vi "change type for single diagram.vi"(8 "error in (no error)":errorcluster, 9 "old type":T1, 10 "new type":T1, 11 "Diagram in":refnum<vi>) -> ()   [LabVIEW 2013]
uses:
  source/tag/Data Type.ctl
  source/tag/tag descriptor.lvclass
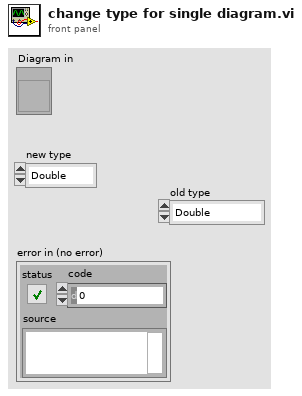
[diagram p1: front panel]
types:
  T1 = typedef "tag bus.lvlib/tag descriptor.lvclass/Data Type.ctl" = enum16{"Double", "Single", "I64", "I32", "I16", "I8", "U64", "U32", "U16", "U8", "Boolean", "String", "Array of Double", "Array of Single", "Array of I64", "Array of I32", "Array of I16", "Array of I8", "Array of U64", "Array of U32", "Array of U16", "Array of U8", "Array of Boolean", "Array of String"}
  T2 = cluster{"VIPath":path, "Menu Name":string, "Selector Name":string}[]
  T3 = cluster{"VIPath":path, "Menu Name":string, "Selector Name":string}
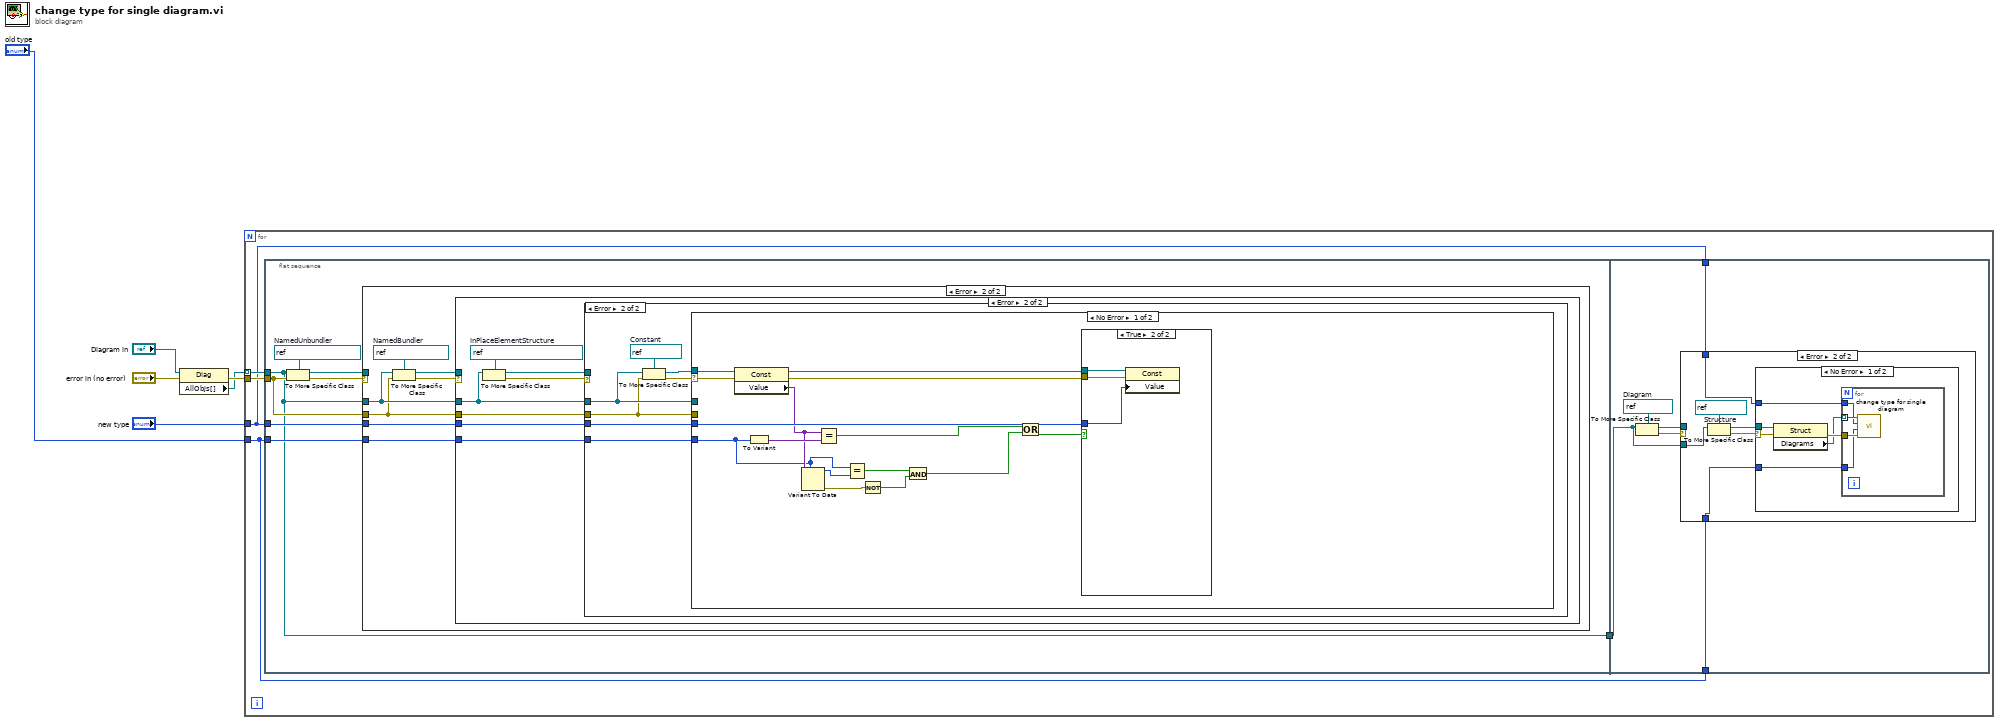
[diagram p0: block diagram]
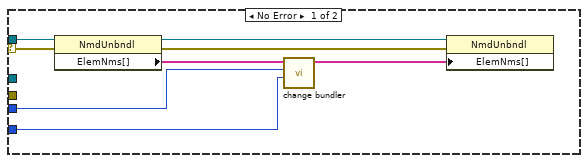
[diagram p2: hidden frame]
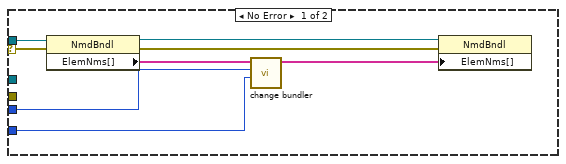
[diagram p3: hidden frame]
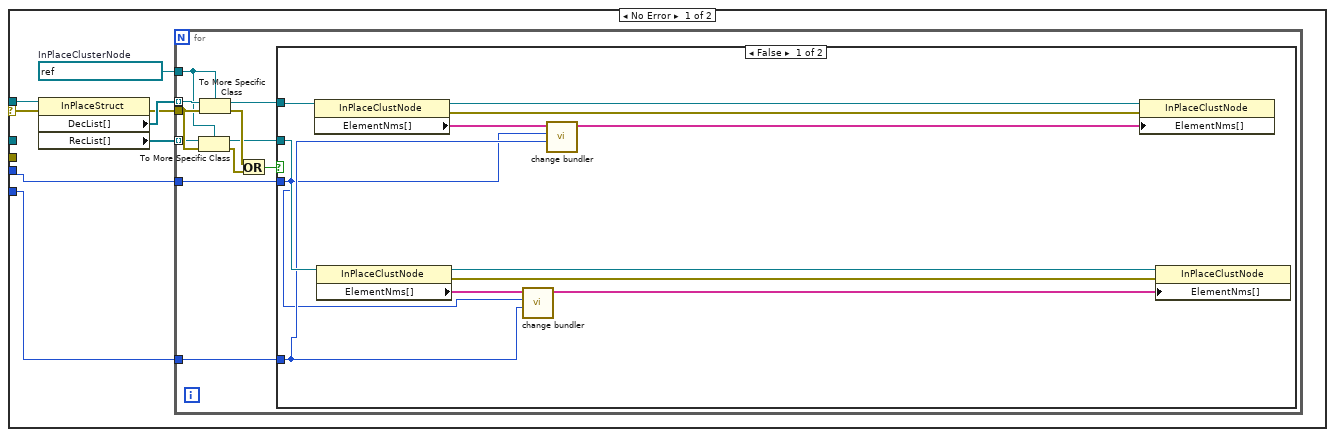
[diagram p4: hidden frame]
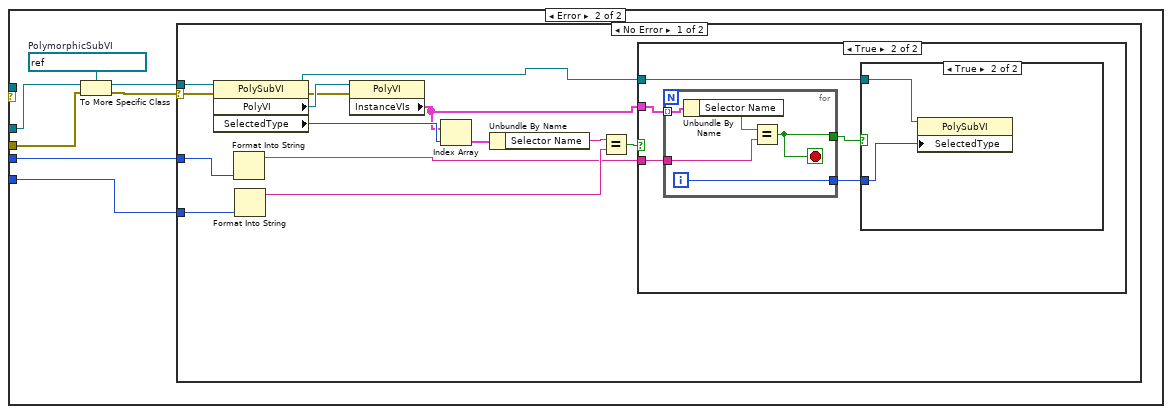
[diagram p7: hidden frame]
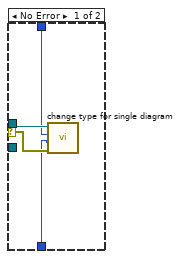
[diagram p11: hidden frame]
diagram:
  n1 = property class="Diag"(reference="Diagram in", error in="error in (no error)") -> (error out=w4:errorcluster, "AllObjs[]"=w3:refnum<vi>[])  [unwired: 1 out]
  n2 = for {
    tunnel: w3 -> [w11] mode=indexing
    tunnel: w4 -> [w10]
    tunnel: "old type" -> [w7]
    tunnel: "new type" -> [w8]
    n3 = flat-sequence {
      tunnel: w11 -> [w12]
      tunnel: w10 -> [w15]
      tunnel: w7 -> [w14]
      tunnel: w8 -> [w13]
      tunnel: [w12] -> w9
      tunnel: w9 -> [w138]
      tunnel: w8 -> [w140]
      tunnel: w7 -> [w139]
      frame #0 {
        w18 = refnum<vi> refnum  # NamedUnbundler
        n4 = To More Specific Class(target class=w18, reference=w12, error in=w15) -> (specific class reference=w16:refnum<vi>, error out=w17:errorcluster)
        n5 = case shown="Error" w17 {
          selector: w17 -> [w25 _]
          tunnel: w16 -> [w26 _]
          tunnel: w12 -> [_ w30]
          tunnel: w15 -> [_ w29]
          tunnel: w14 -> [w20 w28]
          tunnel: w13 -> [w19 w27]
          frame No Error {
            n6 = property class="NmdUnbndl"(reference=w26, error in=w25) -> (reference out=w24:refnum<vi>, error out=w23:errorcluster, "ElemNms[]"=w22:string[])
            n7 = call "change bundler.vi"("old data type"=w20, "new data type"=w19, "ElemNms[]"=w22) -> ("elemnames out"=w21:string[])  [unwired: 8 in]
            n8 = property class="NmdUnbndl"(reference=w24, error in=w23, "ElemNms[]"=w21) -> ()  [unwired: 2 out]
          }
          frame Error {
            w33 = refnum<vi> refnum  # NamedBundler
            n9 = To More Specific Class(target class=w33, reference=w30, error in=w29) -> (specific class reference=w31:refnum<vi>, error out=w32:errorcluster)
            n10 = case shown="Error" w32 {
              selector: w32 -> [w36 _]
              tunnel: w31 -> [w37 _]
              tunnel: w30 -> [_ w42]
              tunnel: w29 -> [_ w45]
              tunnel: w28 -> [w34 w44]
              tunnel: w27 -> [w35 w43]
              frame No Error {
                n11 = property class="NmdBndl"(reference=w37, error in=w36) -> (reference out=w40:refnum<vi>, error out=w39:errorcluster, "ElemNms[]"=w41:string[])
                n12 = call "change bundler.vi"("old data type"=w34, "new data type"=w35, "ElemNms[]"=w41) -> ("elemnames out"=w38:string[])  [unwired: 8 in]
                n13 = property class="NmdBndl"(reference=w40, error in=w39, "ElemNms[]"=w38) -> ()  [unwired: 2 out]
              }
              frame Error {
                w48 = refnum<vi> refnum  # InPlaceElementStructure
                n14 = To More Specific Class(target class=w48, reference=w42) -> (specific class reference=w46:refnum<vi>, error out=w47:errorcluster)  [unwired: 1 in]
                n15 = case shown="Error" w47 {
                  selector: w47 -> [w55 _]
                  tunnel: w46 -> [w56 _]
                  tunnel: w42 -> [_ w81]
                  tunnel: w45 -> [_ w80]
                  tunnel: w44 -> [w49 w83]
                  tunnel: w43 -> [w50 w82]
                  frame No Error {
                    w52 = refnum<vi> refnum  # InPlaceClusterNode
                    n16 = property class="InPlaceStruct"(reference=w56, error in=w55) -> (error out=w53:errorcluster, "DecList[]"=w54:refnum<vi>[], "RecList[]"=w51:refnum<vi>[])  [unwired: 1 out]
                    n17 = for {
                      tunnel: w54 -> [w67] mode=indexing
                      tunnel: w53 -> [w66]
                      tunnel: w52 -> [w64]
                      tunnel: w51 -> [w65] mode=indexing
                      tunnel: w50 -> [w58]
                      tunnel: w49 -> [w57]
                      n18 = To More Specific Class(target class=w64, reference=w65, error in=w66) -> (specific class reference=w59:refnum<vi>, error out=w62:errorcluster)
                      n19 = To More Specific Class(target class=w64, reference=w67, error in=w66) -> (specific class reference=w60:refnum<vi>, error out=w63:errorcluster)
                      n20 = Or(x=w63, y=w62) -> (x .or. y?=w61:bool)
                      n21 = case shown="False" w61 {
                        tunnel: w60 -> [w74 _]
                        tunnel: w59 -> [w75 _]
                        tunnel: w58 -> [w68 _]
                        tunnel: w57 -> [w69 _]
                        frame False {
                          n22 = property class="InPlaceClustNode"(reference=w74) -> (reference out=w79:refnum<vi>, error out=w78:errorcluster, "ElementNms[]"=w71:string[])  [unwired: 1 in]
                          n23 = property class="InPlaceClustNode"(reference=w75) -> (reference out=w76:refnum<vi>, error out=w77:errorcluster, "ElementNms[]"=w73:string[])  [unwired: 1 in]
                          n24 = call "change bundler.vi"("old data type"=w69, "new data type"=w68, "ElemNms[]"=w73) -> ("elemnames out"=w72:string[])  [unwired: 8 in]
                          n25 = call "change bundler.vi"("old data type"=w69, "new data type"=w68, "ElemNms[]"=w71) -> ("elemnames out"=w70:string[])  [unwired: 8 in]
                          n26 = property class="InPlaceClustNode"(reference=w79, error in=w78, "ElementNms[]"=w70) -> ()  [unwired: 2 out]
                          n27 = property class="InPlaceClustNode"(reference=w76, error in=w77, "ElementNms[]"=w72) -> ()  [unwired: 2 out]
                        }
                        frame True {
                          # "shouldnt ever happen if I understand ipestructs"
                        }
                      }
                    }
                  }
                  frame Error {
                    w86 = refnum<vi> refnum  # Constant
                    n28 = To More Specific Class(target class=w86, reference=w81, error in=w80) -> (specific class reference=w84:refnum<vi>, error out=w85:errorcluster)
                    n29 = case shown="No Error" w85 {
                      selector: w85 -> [w100 _]
                      tunnel: w84 -> [w101 _]
                      tunnel: w83 -> [w92 w105]
                      tunnel: w82 -> [w95 w106]
                      tunnel: w81 -> [_ w109]
                      tunnel: w80 -> [_ w110]
                      frame No Error {
                        n30 = property class="Const"(reference=w101, error in=w100) -> (reference out=w97:refnum<vi>, error out=w96:errorcluster, "Value"=w94:variant)
                        n31 = To Variant(anything=w92) -> (Variant=w99:variant)
                        n32 = Variant To Data(type=w92, Variant=w94) -> (data=w93:T1, error out=w90:errorcluster)  [unwired: 1 in]
                        n33 = Equal?(x=w94, y=w99) -> (x = y?=w98:bool)
                        n34 = Equal?(x=w92, y=w93) -> (x = y?=w91:bool)
                        n35 = Not(x=w90) -> (.not. x?=w89:bool)
                        n36 = And(x=w91, y=w89) -> (x .and. y?=w87:bool)
                        n37 = Or(x=w98, y=w87) -> (x .or. y?=w88:bool)
                        n38 = case shown="True" w88 {
                          tunnel: w97 -> [_ w104]
                          tunnel: w96 -> [_ w103]
                          tunnel: w95 -> [_ w102]
                          frame False {
                          }
                          frame True {
                            n39 = property class="Const"(reference=w104, error in=w103, "Value"=w102) -> ()  [unwired: 2 out]
                          }
                        }
                      }
                      frame Error {
                        w111 = refnum<vi> refnum  # PolymorphicSubVI
                        n40 = To More Specific Class(target class=w111, reference=w109, error in=w110) -> (specific class reference=w108:refnum<vi>, error out=w107:errorcluster)
                        n41 = case shown="No Error" w107 {
                          selector: w107 -> [w124 _]
                          tunnel: w108 -> [w125 _]
                          tunnel: w106 -> [w119 _]
                          tunnel: w105 -> [w118 _]
                          frame No Error {
                            n42 = property class="PolySubVI"(reference=w125, error in=w124) -> (reference out=w114:refnum<vi>, error out=w122:errorcluster, "PolyVI"=w123:refnum<vi>, "SelectedType"=w113:i32)
                            n43 = Format Into String(w119) -> (resulting string=w115:string)  [unwired: 3 in, 1 out]
                            n44 = Format Into String(w118) -> (resulting string=w117:string)  [unwired: 3 in, 1 out]
                            n45 = property class="PolyVI"(reference=w123, error in=w122) -> ("InstanceVIs"=w112:T2)  [unwired: 2 out]
                            n46 = Index Array(array=w112, index=w113) -> (element=w121:T3)
                            n47 = Unbundle By Name(w121) -> ("Selector Name"=w120:string)
                            n48 = Equal?(x=w120, y=w117) -> (x = y?=w116:bool)
                            n49 = case shown="True" w116 {
                              tunnel: w112 -> [_ w130]
                              tunnel: w115 -> [_ w129]
                              tunnel: w114 -> [_ w127]
                              frame False {
                              }
                              frame True {
                                n50 = for {
                                tunnel: w130 -> [w137] mode=indexing
                                tunnel: w129 -> [w135]
                                tunnel: [w134] -> w128
                                tunnel: [w133] -> w126
                                i -> [w133]
                                stop <- w134 stop-if-true
                                n51 = Unbundle By Name(w137) -> ("Selector Name"=w136:string)
                                n52 = Equal?(x=w136, y=w135) -> (x = y?=w134:bool)
                                }
                                n53 = case shown="True" w128 {
                                tunnel: w127 -> [_ w132]
                                tunnel: w126 -> [_ w131]
                                frame False {
                                }
                                frame True {
                                n54 = property class="PolySubVI"(reference=w132, "SelectedType"=w131) -> ()  [unwired: 1 in, 2 out]
                                }
                                }
                              }
                            }
                          }
                          frame Error {
                          }
                        }
                      }
                    }
                  }
                }
              }
            }
          }
        }
      }
      frame #1 {
        w143 = refnum<vi> refnum  # Diagram
        n55 = To More Specific Class(target class=w143, reference=w138) -> (specific class reference=w141:refnum<vi>, error out=w142:errorcluster)  [unwired: 1 in]
        n56 = case shown="Error" w142 {
          selector: w142 -> [w146 _]
          tunnel: w141 -> [w147 _]
          tunnel: w140 -> [w145 w149]
          tunnel: w139 -> [w144 w148]
          tunnel: w138 -> [_ w152]
          frame No Error {
            n57 = call "change type for single diagram.vi"("error in (no error)"=w146, "old type"=w144, "new type"=w145, "Diagram in"=w147) -> ()  [unwired: 8 in]
          }
          frame Error {
            w153 = refnum<vi> refnum  # Structure
            n58 = To More Specific Class(target class=w153, reference=w152) -> (specific class reference=w150:refnum<vi>, error out=w151:errorcluster)  [unwired: 1 in]
            n59 = case shown="No Error" w151 {
              selector: w151 -> [w158 _]
              tunnel: w150 -> [w159 _]
              tunnel: w149 -> [w155 _]
              tunnel: w148 -> [w154 _]
              frame No Error {
                n60 = property class="Struct"(reference=w159, error in=w158) -> (error out=w157:errorcluster, "Diagrams"=w156:refnum<vi>[])  [unwired: 1 out]
                n61 = for {
                  tunnel: w157 -> [w163]
                  tunnel: w156 -> [w162] mode=indexing
                  tunnel: w155 -> [w161]
                  tunnel: w154 -> [w160]
                  n62 = call "change type for single diagram.vi"("error in (no error)"=w163, "old type"=w160, "new type"=w161, "Diagram in"=w162) -> ()  [unwired: 8 in]
                }
              }
              frame Error {
              }
            }
          }
        }
      }
    }
  }
